vi "double 2 ms us ns LVConform.vi"(6 "µs":dbl format="%#_12f") -> (0 "sec":i32, 1 "ms":i32, 2 "µs":i32 min=0 max=999, 3 "ns":i32 max=999, 4 "sign":i32)   [LabVIEW 2009, in "CS POLARIS BME DG Client.lvlib"]
uses:
  CS POLARIS BME DG Client.lvlib
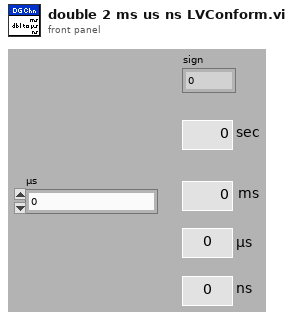
[diagram p1: front panel]
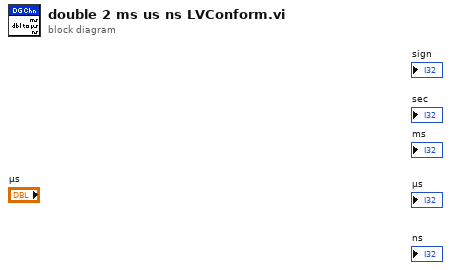
[diagram p0: block diagram]
diagram:
